vi "lift-control.vi"   [LabVIEW 2012, in "Serenity_mk2.lvrbt"]
uses:
  Serenity_mk2.lvrbt
  <vilib>/NXT/Block Support/NXT_ButtonSelector.ctl
  <vilib>/NXT/Hardware/Plugins/Tetrix DC Motor/TetrixDCMotorAddress.ctl
  <vilib>/NXT/Dual Mode Library/Sensors/readNXTButton.vi
  <vilib>/NXT/NXTIO Xnodes/NXTIONodeSubVIs/TETRIX IO Move DC Motors.vi
  <vilib>/NXT/Subs/LVHSConnector.ctl
  <vilib>/NXT/NXTIO Xnodes/AddressXNode/NXTIOAddress.xnode
  MecanumDrive/Mecanum Drive.lvrbt
  <vilib>/NXT/NXTIO Xnodes/NXTIOXNode/NXTIO.xnode
  <vilib>/NXT/LegoClasses/BrickReference/BrickReference.lvclass
types:
  T1 = typedef "NXT_ButtonSelector.ctl" = u16
  T2 = typedef "TetrixDCMotorAddress.ctl" = i32
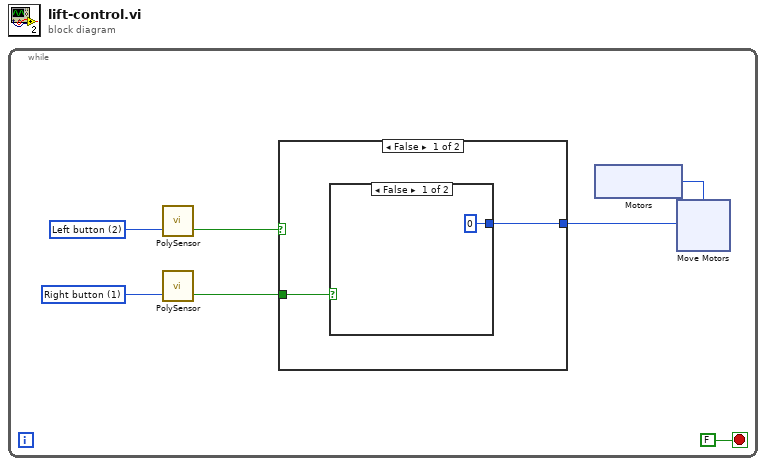
[diagram p0: block diagram]
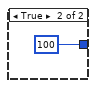
[diagram p2: hidden frame]
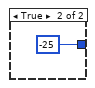
[diagram p3: hidden frame]
diagram:
  n1 = while {
    stop <- FALSE stop-if-true
    w3 = T1 1 items=["Enter button"=3, "Left button"=2, "Right button"=1, "Up Button"=4, "Down Button"=5] ("Button (Enter button)")
    w7 = T1 2 items=["Enter button"=3, "Left button"=2, "Right button"=1, "Up Button"=4, "Down Button"=5] ("Button (Enter button)")
    n2 = call-poly <vilib>:"PolySensor.vi"("Button (Enter button)"=w7) -> ("Yes/No"=w6:bool)  [unwired: 2 in, 1 out]
    n3 = call-poly <vilib>:"PolySensor.vi"("Button (Enter button)"=w3) -> ("Yes/No"=w2:bool)  [unwired: 2 in, 1 out]
    n4 = case shown="False" w6 {
      tunnel: [w16 -25] -> w5
      tunnel: w2 -> [w17 _]
      frame False {
        n5 = case shown="False" w17 {
          tunnel: [0 100] -> w16
          frame False {
          }
          frame True {
          }
        }
      }
      frame True {
      }
    }
    n6 = xnode "Motors"() -> ("Motor"=w4:T2)
    n7 = xnode "Move Motors"("Power/Speed 1"=w5, "Motors"=w4) -> ()  [unwired: 1 in, 1 out]
  }
